vi "PLspectra_mapping.vi"() -> ()   [LabVIEW 2023]
uses:
  <vilib>/Analysis/8numeric.llb/1D Numeric Integration.vi
  <vilib>/Analysis/NI_AALPro.lvlib
panel:
  out "Is XMotion Done1":bool
  out "Is XMotion Done0":bool
  out "millisecond timer value":u32
  in  "DoNOT USE":bool
  out "subarray":i32[](array[numeric])
  out "Number areas":i32=1
  out "Gain description":string[](array[string])
  out "ADC description":string[](array[string])
  out "Gain Number":i32[](array[numeric])
  out "activeYPixels":i32=256
  out "activeXPixels":i32=1024
  out "Is YMotion Done":bool
  out "error out":errorcluster
  out "Identification":string
  out "DeviceKey Out":string
  out "Filename":path caption="Filename Out"
  in  "Save?":bool=TRUE caption="Enable"
  in  "CCD Busy 2":bool caption="CCD Busy"
  in  "stop":bool
  in  "Start Scan":bool caption="Acquire"
  out "Acq Time(ms)":u32
  in  "ShutterOpen":bool
  in  "DisplayArea":i32
  in  "numAreas":i32=2
  out "Gain_supplied":i32
  out "ADC_supplied":i32
  out "DataSize":i32
  in  "Number of Areas :":u16=1 min=1 step=1
  in  "Integration time (ms)":i16
  out "ADC Number":i32[](array[numeric])
  out "FirmwareVersion":string="V1.89  CCD_3000"
  out "nbr of components":i32
  out "CCD DeviceName":string[](array[string])
  out "CCD UniqueID":string[](array[string])
  out "Xloop_iter":i32
  out "Yloop_iter":i32
  out "YPos":i32
  out "XPos":i32
  in  "Xtotalsteps":i32
  in  "Xstep_res (BWD)":i32
  in  "Xstep_res (FWD)":i32
  in  "MotorX":i32
  in  "Wait time (ms) in X":u32
  in  "MotorY":i32
  in  "Ystep_res":i32
  in  "Ytotalsteps":i32
  in  "MinZ":dbl
  out "Intensity Graph":dbl[][](graph)=[[0.0, 960.0, 940.0, 790.0, 950.0, 1030.0, 970.0, 780.0, 990.0, 1010.0, 980.0, 900.0, 1080.0, 950.0, 890.0, 1020.0, 780.0, 1020.0, 950.0, 1180.0], [800.0, 720.0, 880.0, 950.0, 850.0, 960.0, 940.0, 970.0, 830.0, 1050.0, 1140.0, 870.0, 1000.0, 1340.0, 860.0, 1760.0, 980.0, 1900.0, 1120.0, 1650.0], [770.0, 1000.0, 1080.0, 820.0, 880.0, 880.0, 1170.0, 900.0, 750.0, 1110.0, 950.0, 820.0, 780.0, 1510.0, 710.0, 3630.0, 770.0, 4530.0, 1060.0, 4960.0], [570.0, 1040.0, 990.0, 1300.0, 770.0, 940.0, 940.0, 920.0, 1010.0, 920.0, 1030.0, 1170.0, 670.0, 3990.0, 1270.0, 7770.0, 1780.0, 10190.0, 1940.0, 10320.0], [700.0, 2170.0, 720.0, 1070.0, 920.0, 1100.0, 1070.0, 1240.0, 1090.0, 1090.0, 780.0, 2330.0, 1100.0, 9500.0, 2570.0, 13250.0, 3430.0, 18370.0, 4920.0, 15420.0], [1150.0, 4050.0, 870.0, 1990.0, 990.0, 2300.0, 890.0, 2100.0, 890.0, 2030.0, 850.0, 5530.0, 1660.0, 16900.0, 6920.0, 20860.0, 8010.0, 26820.0, 11920.0, 24090.0], [2410.0, 7690.0, 1380.0, 5680.0, 950.0, 5660.0, 1150.0, 6030.0, 1120.0, 5990.0, 1100.0, 13320.0, 4680.0, 23310.0, 12680.0, 30260.0, 15460.0, 37490.0, 20040.0, 32360.0], [3730.0, 11670.0, 3470.0, 10700.0, 2160.0, 11620.0, 2650.0, 13450.0, 1960.0, 16280.0, 3330.0, 24280.0, 9750.0, 29590.0, 19490.0, 39280.0, 25460.0, 44560.0, 28710.0, 38240.0], [5820.0, 13930.0, 7980.0, 15370.0, 5380.0, 18180.0, 6410.0, 22810.0, 6360.0, 28160.0, 9770.0, 34440.0, 18410.0, 42010.0, 27930.0, 47640.0, 36930.0, 51850.0, 36620.0, 38310.0], [10910.0, 18840.0, 11150.0, 20990.0, 10890.0, 24120.0, 12390.0, 32770.0, 15080.0, 36680.0, 20580.0, 46100.0, 28750.0, 52000.0, 34670.0, 57560.0, 43850.0, 55160.0, 43260.0, 39980.0], [15940.0, 18620.0, 14810.0, 27550.0, 16710.0, 32360.0, 19800.0, 43300.0, 25930.0, 49500.0, 33140.0, 57890.0, 36190.0, 59830.0, 45190.0, 66030.0, 50740.0, 62090.0, 48710.0, 40450.0], [18210.0, 21400.0, 20610.0, 32540.0, 22470.0, 41180.0, 26870.0, 55110.0, 36190.0, 59600.0, 45000.0, 71170.0, 49620.0, 77020.0, 54950.0, 77120.0, 60070.0, 65320.0, 47310.0, 41610.0], [19980.0, 27630.0, 24900.0, 39620.0, 30920.0, 51640.0, 41210.0, 64930.0, 48560.0, 75980.0, 58830.0, 80180.0, 62620.0, 87370.0, 65050.0, 89380.0, 67340.0, 71060.0, 52720.0, 42330.0], [22060.0, 37480.0, 29730.0, 46150.0, 36490.0, 61910.0, 51530.0, 75500.0, 57820.0, 89350.0, 70600.0, 94390.0, 78340.0, 96990.0, 80350.0, 100080.0, 79370.0, 79130.0, 55810.0, 45520.0], [30290.0, 47190.0, 34090.0, 53020.0, 45160.0, 73900.0, 63850.0, 88890.0, 70560.0, 101120.0, 83090.0, 103760.0, 86430.0, 106600.0, 95730.0, 104970.0, 86060.0, 78120.0, 60830.0, 48710.0], [38810.0, 59500.0, 41970.0, 66520.0, 54310.0, 87210.0, 76860.0, 101460.0, 84910.0, 110370.0, 96060.0, 118150.0, 97970.0, 118660.0, 105500.0, 102890.0, 92680.0, 80660.0, 66370.0, 49220.0], [44290.0, 65130.0, 55290.0, 74890.0, 65450.0, 93890.0, 85000.0, 113550.0, 95920.0, 123970.0, 110280.0, 127190.0, 107900.0, 124790.0, 109070.0, 100530.0, 93780.0, 73700.0, 66770.0, 49400.0], [55930.0, 72390.0, 63110.0, 87710.0, 79530.0, 109270.0, 102450.0, 128690.0, 113170.0, 131910.0, 117470.0, 139240.0, 122700.0, 128430.0, 115300.0, 94570.0, 90710.0, 67040.0, 64120.0, 46810.0], [68310.0, 81060.0, 70150.0, 94040.0, 87080.0, 115930.0, 110550.0, 136550.0, 122470.0, 143100.0, 130550.0, 141520.0, 133000.0, 121900.0, 118010.0, 88120.0, 91940.0, 60980.0, 61360.0, 41230.0], [76260.0, 81810.0, 83610.0, 90390.0, 95690.0, 107610.0, 122620.0, 130470.0, 133680.0, 139910.0, 142260.0, 148030.0, 139440.0, 133350.0, 117890.0, 103760.0, 83410.0, 75650.0, 56860.0, 51030.0]]
  out "Data":i32[][](graph)
  out "XY Graph":cluster{"X":dbl[], "Y":dbl[]}[](graph)
  out "result":dbl format="%0.4f"
  out "areas :":i32[][](array[numeric])=[[1], [1], [1], [1440], [1032], [1], [1032]]
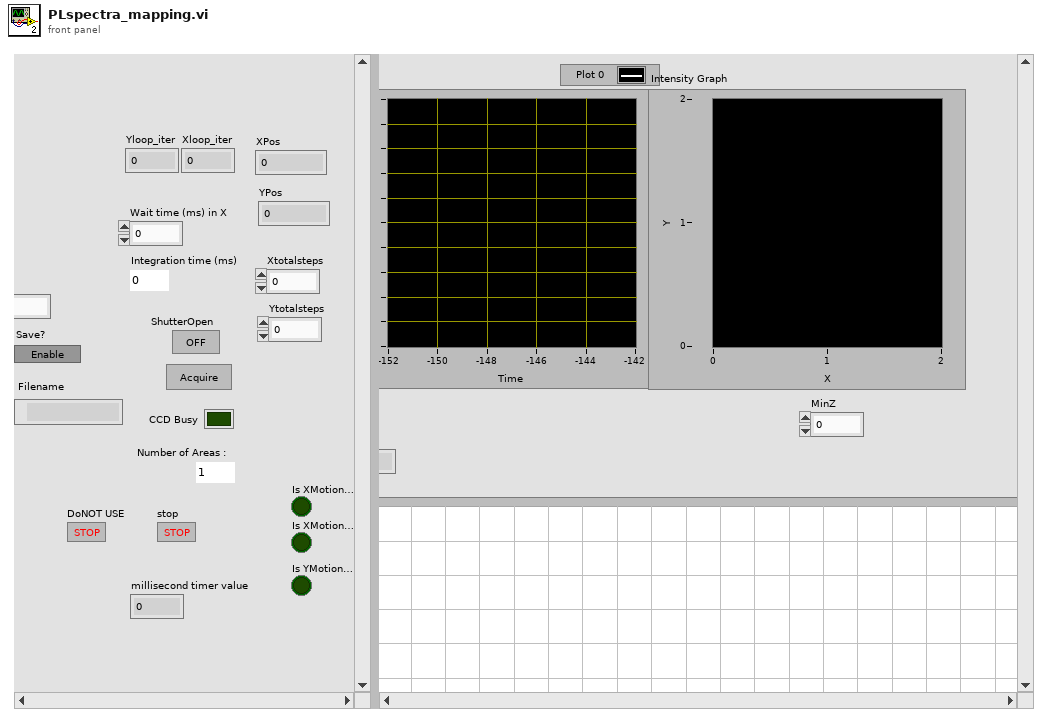
[diagram p1: front panel]
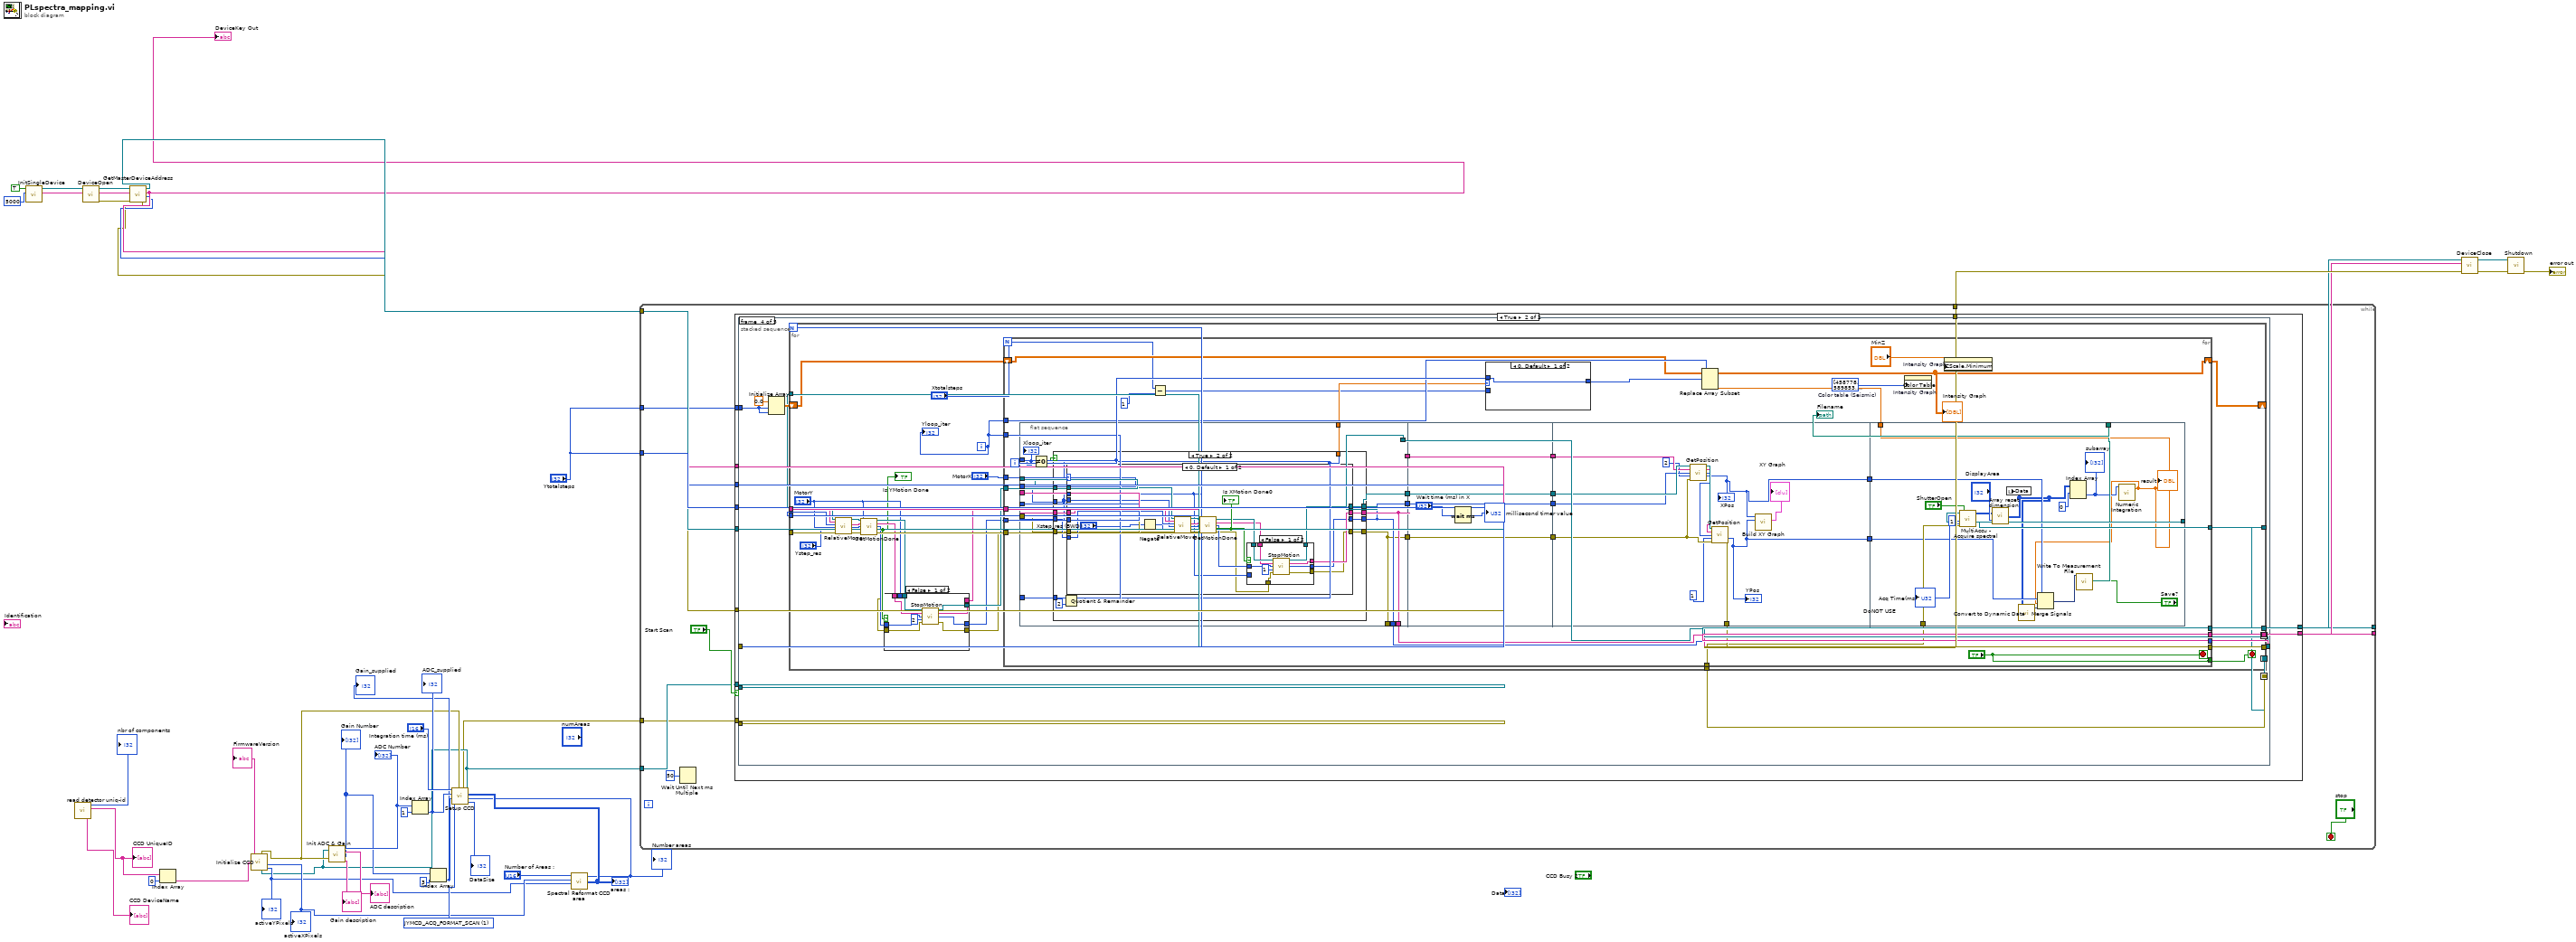
[diagram p0: block diagram]
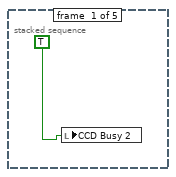
[diagram p3: hidden frame]
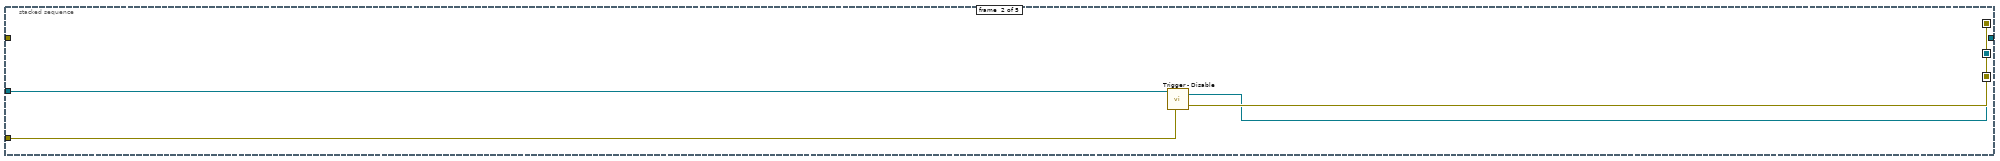
[diagram p4: hidden frame]
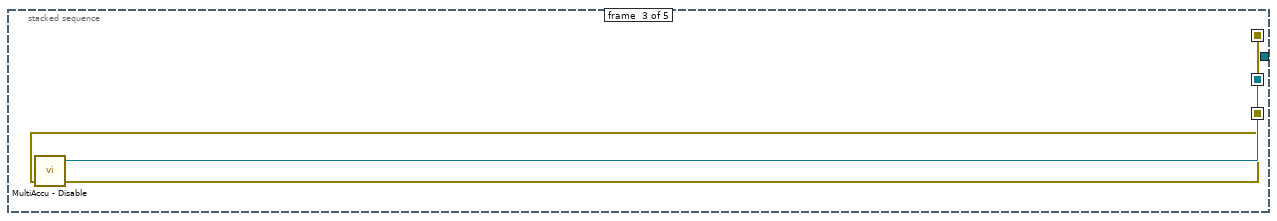
[diagram p5: hidden frame]
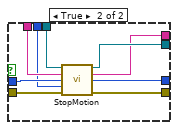
[diagram p6: hidden frame]
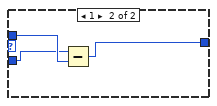
[diagram p7: hidden frame]
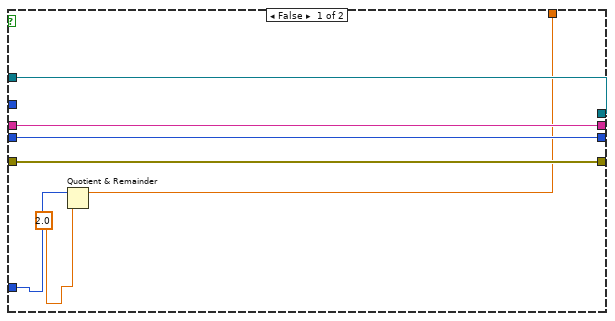
[diagram p8: hidden frame]
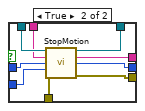
[diagram p9: hidden frame]
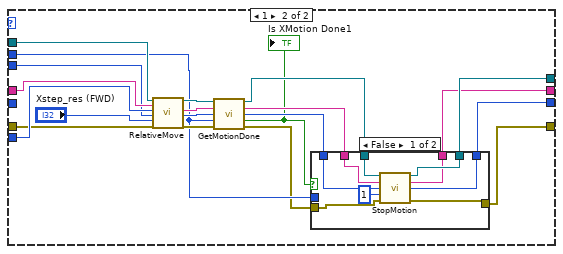
[diagram p10: hidden frame]
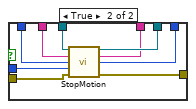
[diagram p11: hidden frame]
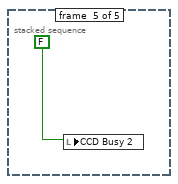
[diagram p12: hidden frame]
diagram:
  w19 = 1 items=["JYMCD_ACQ_FORMAT_IMAGE", "JYMCD_ACQ_FORMAT_SCAN"] ("Acquisition type")
  n1 = call "InitSingleDevice.vi"("msecDelayForDiscovery"=5000, "logging"=TRUE) -> ("DeviceKey Out"=w38:string, "CmdLib Out"=w39:refnum<k24>)  [unwired: 3 in, 1 out]
  n2 = call "read detector uniq-id.vi"() -> ("nbr of components"=→"nbr of components":i32, "UniqueID"=w32:string[], "DeviceName"=→"CCD DeviceName":string[])  [unwired: 3 in, 1 out]
  "CCD UniqueID" <- w32
  n3 = call "DeviceOpen.vi"("DeviceKey In"=w38, "CmdLib In"=w39) -> ("error out"=w42:errorcluster, "DeviceKey Out"=w41:string, "CmdLib Out"=w40:refnum<k24>)  [unwired: 3 in]
  n4 = call "GetMasterDeviceAddress.vi"("error in (no error)"=w42, "DeviceKey In"=w41, "CmdLib In"=w40) -> ("error out"=w5:errorcluster, "Device Address"=w6:i32, "DeviceKey Out"=w7:string, "CmdLib Out"=w8:refnum<k24>)  [unwired: 1 in]
  "DeviceKey Out" <- w7
  n5 = Index Array(array=w32, index=0) -> (element=w30:string)
  n6 = call "Initialize CCD.vi"("Unique id:"=w30) -> ("activeYPixels"=w16:i32, "JYCCDLib.IJYCCDReqd"=w10:refnum<k7>, "activeXPixels"=w17:i32, "sortie d'erreur"=w18:errorcluster, "FirmwareVersion"=→"FirmwareVersion":string)  [unwired: 2 in, 1 out]
  "activeXPixels" <- w17
  "activeYPixels" <- w16
  n7 = call "Init ADC & Gain.vi"("JYCCDLib.IJYCCDReqd"=w10, "input error"=w18) -> ("ADC Number"=w25:i32[], "ADC description"=→"ADC description":string[], "Gain Number"=w22:i32[], "Gain description"=→"Gain description":string[])
  "ADC Number" <- w25
  "Gain Number" <- w22
  n8 = Index Array(array=w25, index=1) -> (element=w23:i32)
  "ADC_supplied" <- w23
  n9 = Index Array(array=w22, index=3) -> (element=w20:i32)
  "Gain_supplied" <- w20
  n10 = call "Spectral Reformat CCD area.vi"("Y Pixels:"=w16, "X Pixels:"=w17, "numAreas"="Number of Areas :") -> ("areas :"=w15:i32[][], "Number areas"=w12:i32)  [unwired: 2 in]
  "areas :" <- w15
  "Number areas" <- w12
  n11 = call "Setup CCD.vi"("numAreas"=w12, "areas :"=w15, "JYCCDLib.IJYCCDReqd"=w10, "entrée d'erreur (pas d'erreur)"=w18, "Acquisition type"=w19, "Gain"=w20, "Select ADC"=w23, "Integration time(ms)"="Integration time (ms)") -> ("DataSize"=→"DataSize":i32, "sortie d'erreur"=w9:errorcluster)
  n12 = while {
    tunnel: w10 -> [w56]
    tunnel: w9 -> [w55]
    tunnel: "Ytotalsteps" -> [w54]
    tunnel: w8 -> [w53]
    tunnel: w7 -> [w52]
    tunnel: w6 -> [w51]
    tunnel: w5 -> [w50]
    tunnel: [w49] -> w4
    tunnel: [w48] -> w3
    tunnel: [w47] -> w2
    tunnel: "Ytotalsteps" -> [w46]
    stop <- "stop" stop-if-true
    n13 = case shown="True" "Start Scan" {
      tunnel: w56 -> [_ w71]
      tunnel: w55 -> [_ w70]
      tunnel: w54 -> [_ w69]
      tunnel: w53 -> [w59 w68]
      tunnel: w52 -> [w58 w67]
      tunnel: w51 -> [_ w66]
      tunnel: w50 -> [w60 w65]
      tunnel: [w60 w64] -> w49
      tunnel: [w58 w63] -> w48
      tunnel: [w59 w62] -> w47
      tunnel: w46 -> [_ w61]
      frame False {
      }
      frame True {
        n14 = stacked-sequence {
          seq-local: [_ w74 _ _ _] -> [_ _ w78 _ _]
          seq-local: [_ w73 _ _ _] -> [_ _ w79 w83 _]
          seq-local: [_ _ w77 _ _] -> [_ _ _ w84 _]
          tunnel: w71 -> [_ w76 _ _ _]
          tunnel: w70 -> [_ w75 _ _ _]
          tunnel: w69 -> [_ _ _ w92 _]
          tunnel: w68 -> [_ _ _ w91 _]
          tunnel: w67 -> [_ _ _ w90 _]
          tunnel: w66 -> [_ _ _ w89 _]
          tunnel: w65 -> [_ _ _ w88 _]
          tunnel: [_ _ _ w87 _] -> w64
          tunnel: [_ _ _ w86 _] -> w63
          tunnel: [_ _ _ w85 _] -> w62
          tunnel: w61 -> [_ _ _ w82 _]
          frame #0 {
            n15 = local write "CCD Busy 2"(TRUE) -> ()
          }
          frame #1 {
            n16 = call "Trigger - Disable.vi"("Error In"=w75, "JYCCDLib.IJYCCDReqd"=w76) -> ("Error Out"=w74:errorcluster, "JYCCDLib.IJYCCDReqd"=w73:refnum<k7>)  [unwired: 4 in]
          }
          frame #2 {
            n17 = call "MultiAccu - Disable.vi"("Error In"=w78, "JYCCDLib.IJYCCDReqd"=w79) -> ("Error Out"=w77:errorcluster)  [unwired: 2 in, 1 out]
          }
          frame #3 {
            n18 = Initialize Array(0.0 ("element"), w82, w82) -> (w80:dbl[][])
            n19 = for {
              N: w92 -> [_]
              tunnel: w91 -> [w118]
              tunnel: w90 -> [w117]
              tunnel: w89 -> [w116]
              tunnel: w88 -> [w115]
              tunnel: [w113] -> w87
              tunnel: [w112] -> w86
              tunnel: [w111] -> w85
              tunnel: w84 -> [w109]
              tunnel: w83 -> [w108]
              shift-right: [w105] -> _
              shift-left: w80 -> [w106]
              i -> [w104]
              stop <- w103 stop-if-true
              n20 = call "RelativeMove.vi"("CmdLib In"=w118, "DeviceKey In"=w117, "Device Address In"=w116, "Motor"="MotorY", "Relative Steps"="Ystep_res", "error in (no error)"=w115) -> ("CmdLib Out"=w122:refnum<k24>, "DeviceKey Out"=w121:string, "Device Address Out"=w120:i32, "error out"=w119:errorcluster)  [unwired: 10 in]
              n21 = call "GetMotionDone.vi"("CmdLib In"=w122, "DeviceKey In"=w121, "Device Address In"=w120, "Motor"="MotorY", "error in (no error)"=w119) -> ("CmdLib Out"=w102:refnum<k24>, "DeviceKey Out"=w100:string, "Device Address Out"=w98:i32, "Is Motion Done"=w93:bool, "error out"=w95:errorcluster)  [unwired: 6 in]
              "Is YMotion Done" <- w93
              n22 = case shown="False" w93 {
                tunnel: [w123 w140] -> w94
                tunnel: [w129 w139] -> w101
                tunnel: [w127 w138] -> w99
                tunnel: [w125 w137] -> w96
                tunnel: w102 -> [w130 w136]
                tunnel: w100 -> [w128 w135]
                tunnel: w98 -> [w126 w134]
                tunnel: "MotorY" -> [_ w133]
                tunnel: w95 -> [w124 w132]
                frame False {
                  n23 = call "StopMotion.vi"("CmdLib In"=w130, "DeviceKey In"=w128, "Device Address In"=w126, "Motor"=2, "error in (no error)"=w124) -> ("CmdLib Out"=w129:refnum<k24>, "DeviceKey Out"=w127:string, "Device Address Out"=w125:i32, "error out"=w123:errorcluster)  [unwired: 7 in]
                }
                frame True {
                  n24 = call "StopMotion.vi"("CmdLib In"=w136, "DeviceKey In"=w135, "Device Address In"=w134, "Motor"=w133, "error in (no error)"=w132) -> ("CmdLib Out"=w139:refnum<k24>, "DeviceKey Out"=w138:string, "Device Address Out"=w137:i32, "error out"=w140:errorcluster)  [unwired: 7 in]
                }
              }
              n25 = for {
                N: "Xtotalsteps" -> [w156]
                tunnel: w101 -> [w176]
                tunnel: w99 -> [w175]
                tunnel: w96 -> [w174]
                tunnel: "MotorX" -> [w141]
                tunnel: w94 -> [w173]
                tunnel: [w169] -> w113
                tunnel: [w172] -> w112
                tunnel: [w170] -> w111
                tunnel: [w171] -> _
                tunnel: w109 -> [w168]
                tunnel: w108 -> [w167]
                tunnel: w104 -> [w162]
                shift-right: [w160] -> w105
                shift-left: w106 -> [w161]
                tunnel: w104 -> [w159]
                tunnel: ["DoNOT USE"] -> w103
                i -> [w163]
                stop <- "DoNOT USE" stop-if-true
                w153 = u32[] [458778, 589853, 655393, 720933, 852008, 917548, 983087, 1114163, 1179703, 1310778, 1376318, 1441858, 1507397, 1572937, 1572940, 1638480, 1638484, 1704023, 1704027, 1769567, 1769570, 1769574, 1769577, 1835117, 1835121, 1835124, 1835128, 1835132, 1769599, 1769603, 1769606, 1769610, 1704078, 1704081, 1638549, 1638553, 1573020, 1573024, 1507491, 1441959, 1441963, 1376430, 1310898, 1245366, 1179834, 1114307, 1048775, 983243, 917711, 786644, 721116, 655584, 524516, 458984, 327917, 196853, 197113, 66045, 511, 1023, 264703, 528383, 792063, 792063, 1121279, 1384959, 1648639, 1912063, 2241279, 2504703, 2768383, 3031807, 3361023, 3624447, 3887871, 4151295, 4480511, 4743935, 5007359, 5270783, 5533951, 5862911, 6126335, 6389759, 6652927, 6981887, 7245055, 7508479, 7771647, 8100351, 8363775, 8626943, 8890111, 9218815, 9481983, 9745151, 10008063, 10336767, 10599935, 10863103, 11126015, 11454719, 11717631, 11980799, 12243711, 12572159, 12835071, 13098239, 13361151, 13689599, 13952511, 14215167, 14478079, 14806527, 15069439, 15332095, 15595007, 15923199, 16186111, 16448511, 16776958, 16776443, 16775671, 16775155, 16774384, 16773868, 16773096, 16772325, 16771553, 16770781, 16770010, 16769238, 16768466, 16767694, 16766923, 16766151, 16765379, 16764608, 16763580, 16762808, 16762037, 16761009, 16760237, 16759210, 16758438, 16757410, 16756382, 16755611, 16754583, 16753555, 16752528, 16751500, 16750728, 16749701, 16748673, 16747389, 16746362, 16745334, 16744306, 16743278, 16741995, 16740967, 16739939, 16738656, 16737628, 16736344, 16735061, 16734033, 16732749, 16731466, 16730438, 16729154, 16727870, 16726862, 16725835, 16724808, 16724037, 16723010, 16721984, 16721213, 16720186, 16719159, 16718389, 16717362, 16716335, 16715308, 16714538, 16713511, 16712484, 16711714, 16580642, 16580642, 16449570, 16318499, 16187427, 15859747, 15728675, 15597603, 15466531, 15269923, 15007779, 14876708, 14680100, 14549028, 14417956, 14090276, 13959204, 13828132, 13565988, 13369380, 13238308, 13041700, 12845092, 12714020, 12517412, 12320804, 12189731, 11993123, 11796515, 11665443, 11468835, 11272227, 11141155, 10944547, 10747938, 10616866, 10420258, 10223650, 10092578, 9895969, 9699361, 9568289, 9371680, 9175072, 9044000, 8847392, 8650783, 8519711, 8323103, 8126494, 7995422, 7798813, 7602205, 7471133, 7274524, 7077916, 6946843, 6750235, 6553626, 6422554, 6225945, 6029337, 5898264, 5701656, 5505047]  # Color table (Seismic)
                n26 = flat-sequence {
                  tunnel: w176 -> [w193]
                  tunnel: w175 -> [w192]
                  tunnel: w174 -> [w191]
                  tunnel: w141 -> [w190]
                  tunnel: w173 -> [w189]
                  tunnel: [w185] -> _
                  tunnel: [w187] -> w172
                  tunnel: [w186] -> w171
                  tunnel: [w188] -> w170
                  tunnel: [w188] -> w149
                  tunnel: [w187] -> w147
                  tunnel: [w186] -> w145
                  tunnel: [w185] -> w143
                  tunnel: w163 -> [w183]
                  tunnel: w159 -> [w182]
                  tunnel: [w181] -> w158
                  tunnel: w149 -> [w295]
                  tunnel: [w295] -> w148
                  tunnel: w147 -> [w294]
                  tunnel: [w294] -> w146
                  tunnel: w145 -> [w293]
                  tunnel: [w293] -> w144
                  tunnel: w143 -> [w292]
                  tunnel: [w292] -> w142
                  tunnel: w148 -> [w308]
                  tunnel: w146 -> [w307]
                  tunnel: w144 -> [w306]
                  tunnel: w142 -> [w304]
                  tunnel: [w298] -> w169
                  tunnel: [w297] -> w165
                  tunnel: [w296] -> w164
                  tunnel: w168 -> [w321]
                  tunnel: w167 -> [w319]
                  tunnel: [w317] -> w166
                  tunnel: w165 -> [w315]
                  tunnel: w164 -> [w314]
                  tunnel: [w312] -> w150
                  frame #0 {
                    n27 = Not Equal To 0?(x=w183) -> (x != 0?=w184:bool)
                    n28 = case shown="True" w184 {
                      tunnel: w193 -> [w200 w212]
                      tunnel: w192 -> [w199 w211]
                      tunnel: w191 -> [w198 w210]
                      tunnel: w190 -> [_ w204]
                      tunnel: w189 -> [w197 w209]
                      tunnel: [w197 w208] -> w185
                      tunnel: [w199 w207] -> w187
                      tunnel: [w198 w206] -> w186
                      tunnel: [w200 w205] -> w188
                      tunnel: w182 -> [w196 w203]
                      tunnel: [w195 w202] -> w181
                      frame False {
                        n29 = Quotient & Remainder(x=w196, y=2.0) -> (x-y*floor(x/y)=w195:dbl)  [unwired: 1 out]
                      }
                      frame True {
                        n30 = Quotient & Remainder(x=w203, y=2) -> (x-y*floor(x/y)=w202:i32)  [unwired: 1 out]
                        n31 = case shown="0, Default" w202 {
                          tunnel: w212 -> [w229 w268]
                          tunnel: w211 -> [w228 w267]
                          tunnel: w210 -> [w227 w266]
                          tunnel: w204 -> [w223 w265]
                          tunnel: w204 -> [w215 w255]
                          tunnel: w209 -> [w226 w262]
                          tunnel: [w213 w253] -> w208
                          tunnel: [w218 w258] -> w207
                          tunnel: [w216 w256] -> w206
                          tunnel: [w220 w260] -> w205
                          tunnel: w204 -> [_ _]
                          frame 0, Default {
                            n32 = Negate(x="Xstep_res (BWD)") -> (-x=w224:i32)
                            n33 = call "RelativeMove.vi"("CmdLib In"=w229, "DeviceKey In"=w228, "Device Address In"=w227, "Motor"=w223, "Relative Steps"=w224, "error in (no error)"=w226) -> ("CmdLib Out"=w232:refnum<k24>, "DeviceKey Out"=w233:string, "Device Address Out"=w231:i32, "error out"=w230:errorcluster)  [unwired: 10 in]
                            n34 = call "GetMotionDone.vi"("CmdLib In"=w232, "DeviceKey In"=w233, "Device Address In"=w231, "Motor"=w215, "error in (no error)"=w230) -> ("CmdLib Out"=w221:refnum<k24>, "DeviceKey Out"=w219:string, "Device Address Out"=w217:i32, "Is Motion Done"=w222:bool, "error out"=w214:errorcluster)  [unwired: 6 in]
                            "Is XMotion Done0" <- w222
                            n35 = case shown="False" w222 {
                              tunnel: w221 -> [w241 w251]
                              tunnel: [w240 w250] -> w220
                              tunnel: w219 -> [w239 w249]
                              tunnel: [w238 w248] -> w218
                              tunnel: w217 -> [w236 w247]
                              tunnel: [w237 w246] -> w216
                              tunnel: w215 -> [_ w245]
                              tunnel: w214 -> [w235 w244]
                              tunnel: [w234 w243] -> w213
                              frame False {
                                n36 = call "StopMotion.vi"("CmdLib In"=w241, "DeviceKey In"=w239, "Device Address In"=w236, "Motor"=1, "error in (no error)"=w235) -> ("CmdLib Out"=w240:refnum<k24>, "DeviceKey Out"=w238:string, "Device Address Out"=w237:i32, "error out"=w234:errorcluster)  [unwired: 7 in]
                              }
                              frame True {
                                n37 = call "StopMotion.vi"("CmdLib In"=w251, "DeviceKey In"=w249, "Device Address In"=w247, "Motor"=w245, "error in (no error)"=w244) -> ("CmdLib Out"=w250:refnum<k24>, "DeviceKey Out"=w248:string, "Device Address Out"=w246:i32, "error out"=w243:errorcluster)  [unwired: 7 in]
                              }
                            }
                          }
                          frame 1 {
                            n38 = call "RelativeMove.vi"("CmdLib In"=w268, "DeviceKey In"=w267, "Device Address In"=w266, "Motor"=w265, "Relative Steps"="Xstep_res (FWD)", "error in (no error)"=w262) -> ("CmdLib Out"=w264:refnum<k24>, "DeviceKey Out"=w263:string, "Device Address Out"=w269:i32, "error out"=w270:errorcluster)  [unwired: 10 in]
                            n39 = call "GetMotionDone.vi"("CmdLib In"=w264, "DeviceKey In"=w263, "Device Address In"=w269, "Motor"=w255, "error in (no error)"=w270) -> ("CmdLib Out"=w261:refnum<k24>, "DeviceKey Out"=w259:string, "Device Address Out"=w257:i32, "Is Motion Done"=w252:bool, "error out"=w254:errorcluster)  [unwired: 6 in]
                            "Is XMotion Done1" <- w252
                            n40 = case shown="False" w252 {
                              tunnel: w261 -> [w279 w289]
                              tunnel: [w280 w288] -> w260
                              tunnel: w259 -> [w278 w287]
                              tunnel: [w277 w286] -> w258
                              tunnel: w257 -> [w276 w285]
                              tunnel: [w275 w284] -> w256
                              tunnel: w255 -> [_ w283]
                              tunnel: w254 -> [w272 w282]
                              tunnel: [w273 w281] -> w253
                              frame False {
                                n41 = call "StopMotion.vi"("CmdLib In"=w279, "DeviceKey In"=w278, "Device Address In"=w276, "Motor"=1, "error in (no error)"=w272) -> ("CmdLib Out"=w280:refnum<k24>, "DeviceKey Out"=w277:string, "Device Address Out"=w275:i32, "error out"=w273:errorcluster)  [unwired: 7 in]
                              }
                              frame True {
                                n42 = call "StopMotion.vi"("CmdLib In"=w289, "DeviceKey In"=w287, "Device Address In"=w285, "Motor"=w283, "error in (no error)"=w282) -> ("CmdLib Out"=w288:refnum<k24>, "DeviceKey Out"=w286:string, "Device Address Out"=w284:i32, "error out"=w281:errorcluster)  [unwired: 7 in]
                              }
                            }
                          }
                        }
                      }
                    }
                    "Xloop_iter" <- w183
                  }
                  frame #1 {
                    n43 = Wait (ms)(milliseconds to wait="Wait time (ms) in X") -> (millisecond timer value=→"millisecond timer value":u32)
                  }
                  frame #2 {
                    n44 = call "GetPosition.vi"("CmdLib In"=w308, "DeviceKey In"=w307, "Device Address In"=w306, "Motor"=2, "error in (no error)"=w304) -> ("CmdLib Out"=w303:refnum<k24>, "DeviceKey Out"=w302:string, "Device Address Out"=w301:i32, "Position"=w296:i32)  [unwired: 6 in, 1 out]
                    "XPos" <- w296
                    n45 = call "GetPosition.vi"("CmdLib In"=w303, "DeviceKey In"=w302, "Device Address In"=w301, "Motor"=1, "error in (no error)"=w304) -> ("Position"=w297:i32, "error out"=w298:errorcluster)  [unwired: 6 in, 3 out]
                    "YPos" <- w297
                    n46 = call "Build XY Graph"("Y Input"=w297, "X Input"=w296) -> ("XY Graph"=→"XY Graph":cluster{"X":dbl[], "Y":dbl[]}[])  [unwired: 8 in, 1 out]
                  }
                  frame #3 {
                    n47 = call "MultiAccu - Acquire spectral.vi"("error in"=w321, "Accumulations:"=u16 1, "ShutterOpen"="ShutterOpen", "JYCCDLib.IJYCCDReqd"=w319) -> ("Acq Time(ms)"=→"Acq Time(ms)":u32, "Array Out"=w324:i32[][][])  [unwired: 1 out]
                    n48 = call "Array reset dimension.vi"("Area Number"="DisplayArea", "Array In"=w324) -> ("Array Out"=w311:i32[][])
                    n49 = local write "Data"(w311) -> ()
                    n50 = call "Convert to Dynamic Data"("2D Array"=w311) -> ("Dynamic Data Type"=w310:dynamicdata)  [unwired: 3 in]
                    n51 = Index Array(array=w311, index (row)=0) -> (element=w313:i32[])  [unwired: 1 in]
                    "subarray" <- w313
                    n52 = call-poly <vilib>:"Numeric Integration.vi"("Input Array"=w313) -> ("result"=w312:dbl)  [unwired: 2 in, 1 out]
                    "result" <- w312
                    n53 = Merge Signals(w314, w315, w312, w310) -> (w316:dynamicdata)
                    n54 = call "Write To Measurement File"("Signals"=w316, "Enable"="Save?") -> ("Filename Out"=w317:path)  [unwired: 15 in, 2 out]
                  }
                }
                n55 = Subtract(x=w156, y=1) -> (x-y=w154:i32)
                n56 = case shown="0, Default" w158 {
                  tunnel: w163 -> [w177 w179]
                  tunnel: [w177 w180] -> w157
                  tunnel: w154 -> [_ w178]
                  frame 0, Default {
                  }
                  frame 1 {
                    n57 = Subtract(x=w178, y=w179) -> (x-y=w180:i32)
                  }
                }
                n58 = Replace Array Subset(array=w161, new element=w150, index (row)=w157, index (col)=w162) -> (w160:dbl[][])
                "Intensity Graph" <- w160
                n59 = property on="Intensity Graph" class="IntGraph (strict)"("Color Table"=w153) -> ()  [unwired: 2 in, 2 out]
                n60 = property on="Intensity Graph" class="IntGraph (strict)"("ZScale.Minimum"="MinZ") -> ()  [unwired: 2 in, 2 out]
                "Filename" <- w166
              }
              "Yloop_iter" <- w104
            }
          }
          frame #4 {
            n61 = local write "CCD Busy 2"(FALSE) -> ()
          }
        }
      }
    }
  }
  n62 = Wait Until Next ms Multiple(millisecond multiple=u32 50 ("n millisecondes")) -> ()  [unwired: 1 out]
  n63 = call "DeviceClose.vi"("error in (no error)"=w4, "DeviceKey In"=w3, "CmdLib In"=w2) -> ("error out"=w35:errorcluster, "CmdLib Out"=w36:refnum<k24>)  [unwired: 2 in, 1 out]
  n64 = call "Shutdown.vi"("error in (no error)"=w35, "CmdLib In"=w36) -> ("error out"=→"error out":errorcluster)  [unwired: 4 in, 1 out]
